vi "UpdateActualDepsOfLibraries.vi"(8 "error in (no error)":errorcluster, 9 "Status Indicator Ref":refnum<vi>, 10 "Lvlib paths":path[](array[path]), 11 "CLI in":refnum<class "CLI.lvclass">) -> (0 "error out":errorcluster, 3 "CLI out":refnum<class "CLI.lvclass">)   [LabVIEW 2019, in "DepsWatch.lvlib"]
uses:
  DepsWatch.lvlib
  <vilib>/Wiresmith Technology/G CLI/CLI Class/CLI.lvclass
  <vilib>/Utility/config.llb/NI_LVConfig.lvlib
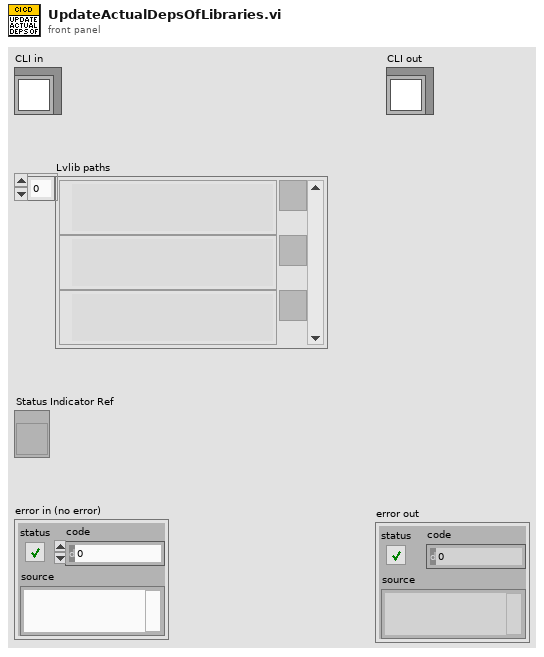
[diagram p1: front panel]
types:
  T1 = typedef "NI_LVConfig.lvlib/Config Data RefNum.ctl" = refnum<k1>
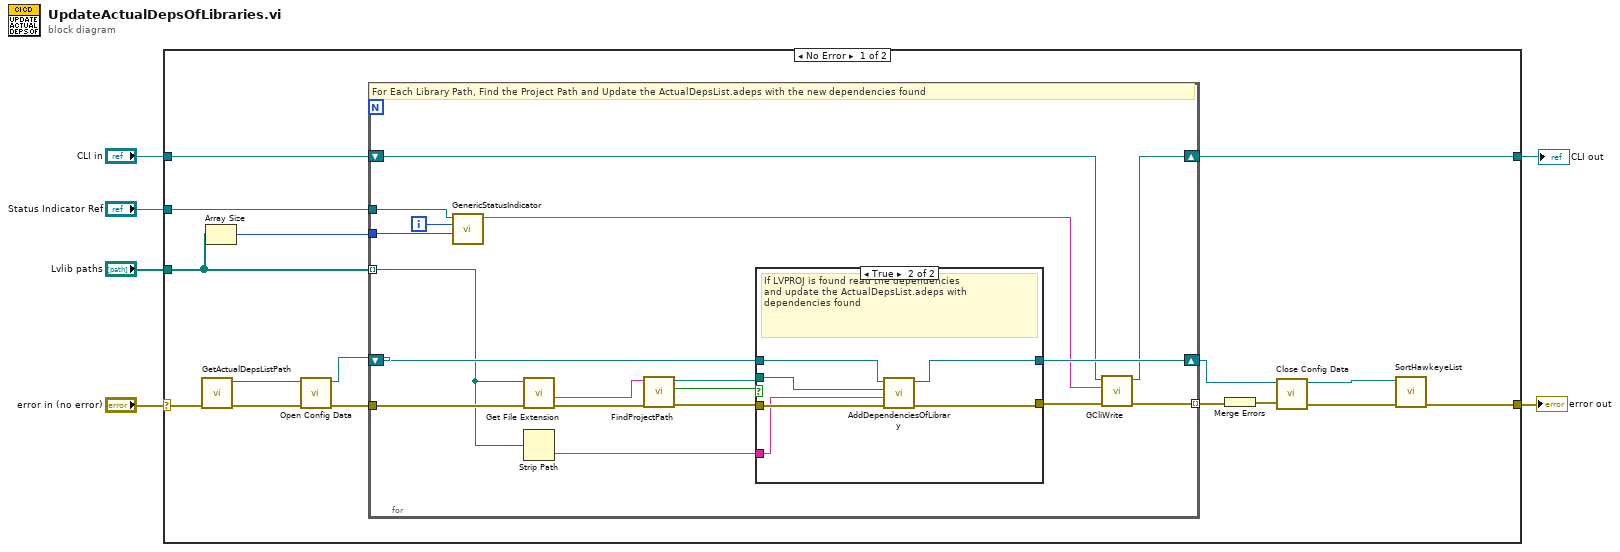
[diagram p0: block diagram]
diagram:
  n1 = case shown="No Error" "error in (no error)" {
    selector: "error in (no error)" -> [w11 w50]
    tunnel: "Status Indicator Ref" -> [w22 _]
    tunnel: [w7 w50] -> w5
    tunnel: [w21 w49] -> w4
    tunnel: "CLI in" -> [w20 w49]
    tunnel: "Lvlib paths" -> [w15 _]
    frame No Error {
      n2 = call "GetActualDepsListPath.vi"("error in (no error)"=w11) -> ("error out"=w19:errorcluster, "ActualDepsListPath"=w18:path)  [unwired: 9 in]
      n3 = Array Size(array=w15) -> (size(s)=w16:i32)
      n4 = call <vilib>:"Open Config Data.vi"("error in (no error)"=w19, "configuration file path"=w18) -> ("error out"=w10:errorcluster, "refnum"=w17:T1)  [unwired: 7 in, 1 out]
      n5 = for {
        tunnel: w10 -> [w40]
        tunnel: w15 -> [w24] mode=indexing
        tunnel: [w29] -> w12 mode=indexing
        shift-right: [w34] -> w14
        shift-left: w17 -> [w35]
        tunnel: w16 -> [w33]
        shift-right: [w28] -> w21
        shift-left: w20 -> [w26]
        tunnel: w22 -> [w31]
        i -> [w32]
        # "For Each Library Path, Find the Project Path and Update the ActualDepsList.adeps with the new dependencies found"
        n6 = call "GenericStatusIndicator.vi"("Total"=w33, "Current Iteration"=w32, "Status Indicator Ref In"=w31) -> ("CLI Status to Print"=w27:string)  [unwired: 8 in]
        n7 = call <vilib>:"Get File Extension.vi"("error in (no error)"=w40, "file"=w24) -> ("error out"=w39:errorcluster, "filename without extension"=w25:string)  [unwired: 5 in, 3 out]
        n8 = Strip Path(path=w24) -> (name=w23:string)  [unwired: 1 out]
        n9 = call "FindProjectPath.vi"("error in (no error)"=w39, "Library/Class Name"=w25) -> ("error out"=w37:errorcluster, "Found?"=w38:bool, "Project Path"=w36:path)  [unwired: 7 in]
        n10 = case shown="True" w38 {
          tunnel: w37 -> [w42 w47]
          tunnel: [w42 w46] -> w30
          tunnel: w36 -> [_ w48]
          tunnel: w35 -> [w41 w45]
          tunnel: [w41 w44] -> w34
          tunnel: w23 -> [_ w43]
          frame False {
            # "If the Project path is not found ignore updating the ActualDepsList.adeps"
          }
          frame True {
            # "If LVPROJ is found read the dependencies \nand update the ActualDepsList.adeps with dependencies found"
            n11 = call "AddDependenciesOfLibrary.vi"("error in (no error)"=w47, "LibraryName"=w43, "Project Path"=w48, "Config Refnum in"=w45) -> ("error out"=w46:errorcluster, "Config Refnum out"=w44:T1)  [unwired: 4 in, 2 out]
          }
        }
        n12 = call "GCliWrite.vi"("error in (no error)"=w30, "Text to Write"=w27, "CLI in"=w26) -> ("error out"=w29:errorcluster, "CLI out"=w28:refnum<class "CLI.lvclass">)  [unwired: 7 in]
      }
      n13 = Merge Errors(w12) -> (w13:errorcluster)
      n14 = call <vilib>:"Close Config Data.vi"("error in (no error)"=w13, "refnum"=w14) -> ("error out"=w8:errorcluster, "file path"=w9:path)  [unwired: 8 in]
      n15 = call "SortHawkeyeList.vi"("error in (no error)"=w8, "Hawkeye File Path"=w9) -> ("error out"=w7:errorcluster)  [unwired: 8 in, 1 out]
    }
    frame Error {
    }
  }
  "error out" <- w5
  "CLI out" <- w4
